vi "ignore error.vi"(6 "error code":i32, 8 "error in":errorcluster) -> (0 "error out":errorcluster, 4 "error found?":bool)   [LabVIEW 2010, in "common.lvlib"]
uses:
  common.lvlib
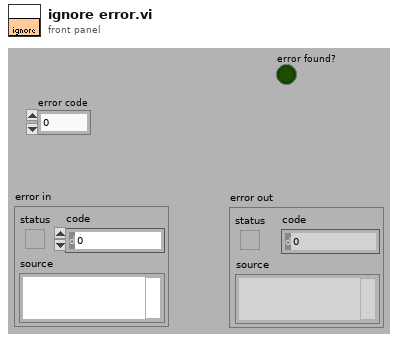
[diagram p1: front panel]
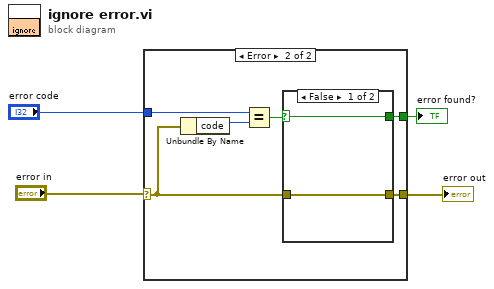
[diagram p0: block diagram]
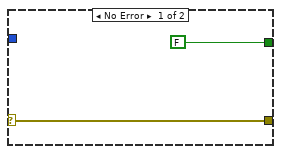
[diagram p2: hidden frame]
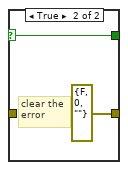
[diagram p3: hidden frame]
diagram:
  n1 = case shown="Error" "error in" {
    selector: "error in" -> [w6 w9]
    tunnel: [w6 w8] -> w3
    tunnel: "error code" -> [_ w11]
    tunnel: [FALSE w7] -> w1
    frame No Error {
    }
    frame Error {
      n2 = Unbundle By Name(w9) -> ("code"=w12:i32)
      n3 = Equal?(x=w11, y=w12) -> (x = y?=w10:bool)
      n4 = case shown="False" w10 {
        selector: w10 -> [w13 w15]
        tunnel: w9 -> [w14 _]
        tunnel: [w14 errorcluster {"status"=FALSE, "code"=0, "source"=""} ("error IO")] -> w8
        tunnel: [w13 w15] -> w7
        frame False {
        }
        frame True {
          # "clear the \nerror"
        }
      }
    }
  }
  "error out" <- w3
  "error found?" <- w1
